vi "Get-action-from-sequence.vi"(5 "Sequence index in":i32, 7 "Motor index":i32, 8 "error in (no error)":errorcluster, 11 "Available motors in":refnum<class "Motor-assembly.lvclass">) -> (0 "error out":errorcluster, 2 "Action":refnum<class "Action.lvclass">, 3 "Available motors out":refnum<class "Motor-assembly.lvclass">, 4 "Sequence index":i32)   [LabVIEW 2013, in "PowderDeposition.lvlib" / "Motor-assembly.lvclass"]
uses:
  Motor-assembly.lvclass
  Action/Action.lvclass
  Motor-assembly.lvclass/Motor-assembly.ctl
  Motor/Motor.lvclass
  Sequence/Action-sequence.lvclass
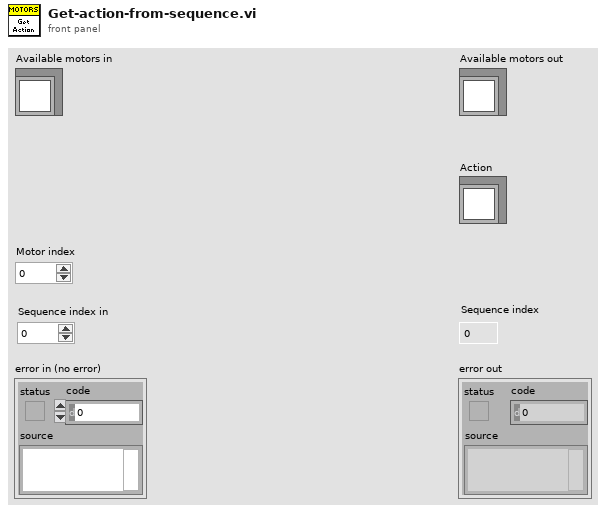
[diagram p1: front panel]
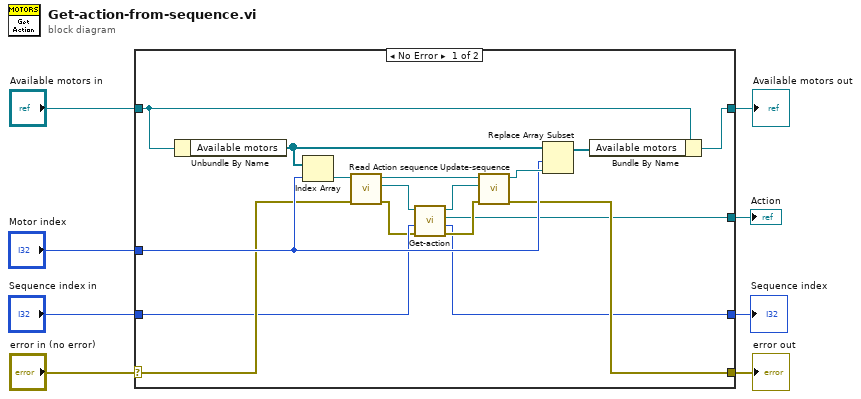
[diagram p0: block diagram]
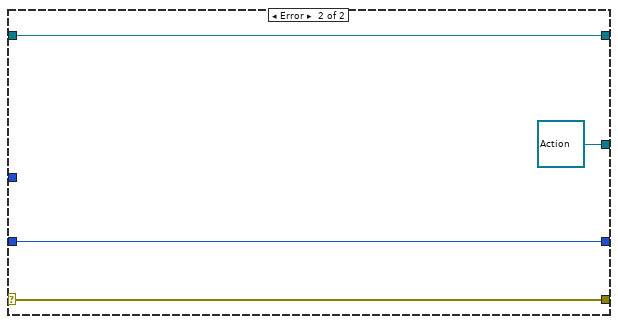
[diagram p2: hidden frame]
diagram:
  n1 = case shown="No Error" "error in (no error)" {
    selector: "error in (no error)" -> [w17 w29]
    tunnel: [w16 w29] -> w7
    tunnel: [w20 w28] -> w5
    tunnel: "Available motors in" -> [w21 w28]
    tunnel: "Motor index" -> [w19 _]
    tunnel: "Sequence index in" -> [w11 w27]
    tunnel: [w12 w27] -> w2
    tunnel: [w9 refnum<class "Action.lvclass"> refnum ("Action")] -> w1
    frame No Error {
      n2 = Unbundle By Name(w21) -> ("Available motors"=w18:refnum<class "Motor.lvclass">[])
      n3 = Index Array(array=w18, index=w19) -> (element=w23:refnum<class "Motor.lvclass">)
      n4 = call-dynamic "Read Action sequence.vi"("error in (no error)"=w17, "Motor in"=w23) -> ("error out"=w10:errorcluster, "Sequence.lvclass"=w15:refnum<class "Action-sequence.lvclass">, "Motor out"=w24:refnum<class "Motor.lvclass">)  [unwired: 7 in]
      n5 = call "Get-action.vi"("error in (no error)"=w10, "Position in"=w11, "Sequence in"=w15) -> ("error out"=w13:errorcluster, "Position"=w12:i32, "Action"=w9:refnum<class "Action.lvclass">, "Sequence out"=w14:refnum<class "Action-sequence.lvclass">)  [unwired: 5 in]
      n6 = call-dynamic "Update-sequence.vi"("error in (no error)"=w13, "Sequence"=w14, "Motor in"=w24) -> ("error out"=w16:errorcluster, "Motor out"=w25:refnum<class "Motor.lvclass">)  [unwired: 7 in]
      n7 = Replace Array Subset(array=w18, new element=w25, index=w19) -> (w22:refnum<class "Motor.lvclass">[])
      n8 = Bundle By Name(cluster=w21, "Available motors"=w22) -> (w20:refnum<class "Motor-assembly.lvclass">)
    }
    frame Error {
    }
  }
  "error out" <- w7
  "Available motors out" <- w5
  "Sequence index" <- w2
  "Action" <- w1
